vi "Write Controller Object.vi"(6 "Device Information":T1={"System Hardware Reference"=refnum, "Device Information"={"Resource"="", "Vendor Name"="", "Product Name"="", "Product ID"=0, "Serial Number"="", "Device Class"="", "System Start Time"=timestamp(0 s since 1904-01-01), "Current Time"=timestamp(0 s since 1904-01-01), "Time Zone"="", "Firmware Revision"="", "Image Title"="", "Image Version"="", "System Status"="", "Credential type"=enum."None/Unlocked", "User Added"=FALSE}, "Primary Network Adapter"={"IP Address"="", "MAC Address"="", "IP Address Request Mode"=1, "SubnetMask"="", "Gateway"="", "DNS Server"="", "Adapter Mode"=1, "Adapter Type"=1}, "Secondary Network Adapters"=[]} {"Primary Network Adapter"."IP Address Request Mode" items=["Static"=1, "DHCP/Link Local"=2, "Link-Local Only"=4, "DHCP Only"=8]; "Primary Network Adapter"."Adapter Type" items=["Ethernet"=1, "WLAN"=2]; "Primary Network Adapter"."Adapter Mode" items=["Disabled"=1, "TCP/IP Ethernet"=2, "Deterministic"=4, "EtherCAT"=8, "TCP/IP WLAN Connect"=32, "TCP/IP WLAN Create"=64]; "Secondary Network Adapters"."IP Address Request Mode" items=["Static"=1, "DHCP/Link Local"=2, "Link-Local Only"=4, "DHCP Only"=8]; "Secondary Network Adapters"."Adapter Type" items=["Disabled"=1, "TCP/IP Ethernet"=2, "Deterministic"=4, "EtherCAT"=8, "TCP/IP WLAN Connect"=32, "TCP/IP WLAN Create"=64]; "Secondary Network Adapters"."Adapter Mode" items=["Disabled"=1, "TCP/IP Ethernet"=2, "Deterministic"=4, "EtherCAT"=8, "TCP/IP WLAN Connect"=32, "TCP/IP WLAN Create"=64]; "Device Information"."Product ID" format="%.0x"}, 8 "error in":errorcluster, 9 "Remote Chassis":refnum<class "Chassis.lvclass">[](array[class]), 10 "Local Chassis":refnum<class "Chassis.lvclass">, 11 "Controller in":refnum<class "Controller.lvclass">) -> (0 "error out":errorcluster, 3 "Controller out":refnum<class "Controller.lvclass">)   [LabVIEW 2015, in "SMI.lvlib" / "Controller.lvclass"]
uses:
  Controller.lvclass
  Controls/NetworkDevice.ctl
  Controls/DeviceInformation.ctl
  Controls/NetworkAdapterSettings.ctl
  Chassis/Chassis.lvclass
  Controller.lvclass/Controller.ctl
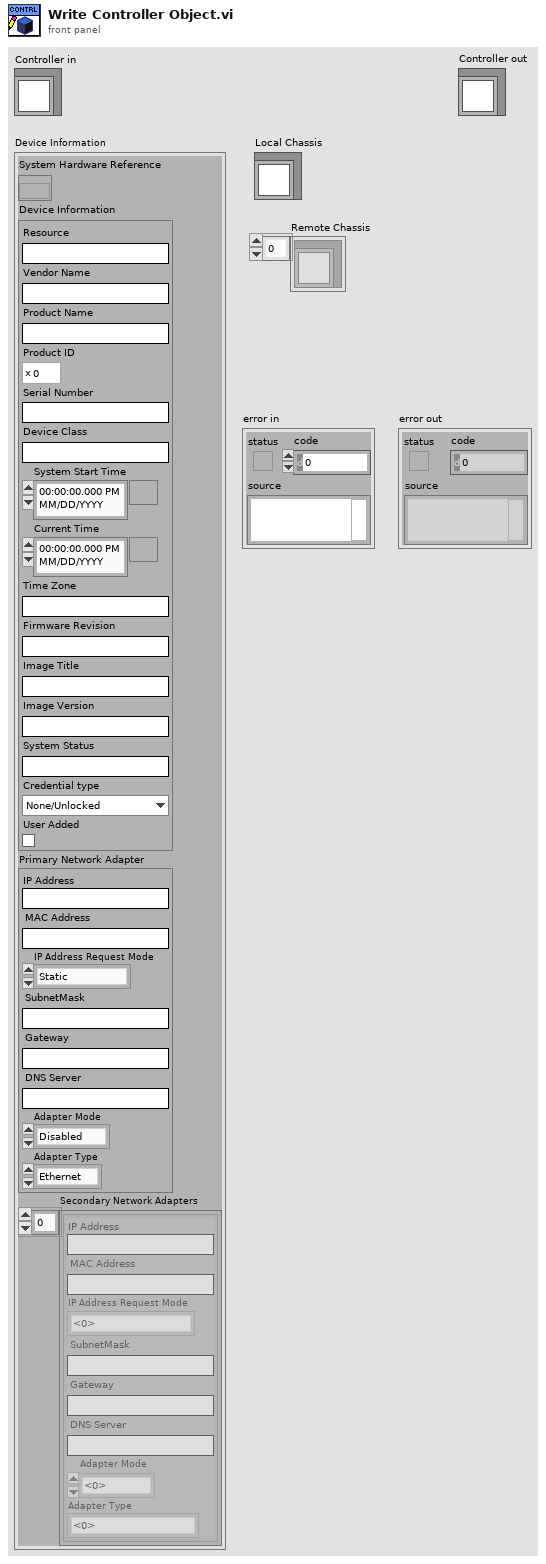
[diagram p1: front panel]
types:
  T1 = typedef "SMI.lvlib/Controller.lvclass/NetworkDevice.ctl" = cluster{"System Hardware Reference":refnum<k20>, "Device Information":T2, "Primary Network Adapter":T3, "Secondary Network Adapters":T3[]}
  T2 = typedef "SMI.lvlib/Controller.lvclass/DeviceInformation.ctl" = cluster{"Resource":string, "Vendor Name":string, "Product Name":string, "Product ID":u32, "Serial Number":string, "Device Class":string, "System Start Time":timestamp, "Current Time":timestamp, "Time Zone":string, "Firmware Revision":string, "Image Title":string, "Image Version":string, "System Status":string, "Credential type":enum16{"None/Unlocked", "FTP Password", "NIAuth Credentials"}, "User Added":bool}
  T3 = typedef "SMI.lvlib/Controller.lvclass/NetworkAdapterSettings.ctl" = cluster{"IP Address":string, "MAC Address":string, "IP Address Request Mode":u32, "SubnetMask":string, "Gateway":string, "DNS Server":string, "Adapter Mode":u32, "Adapter Type":u32}
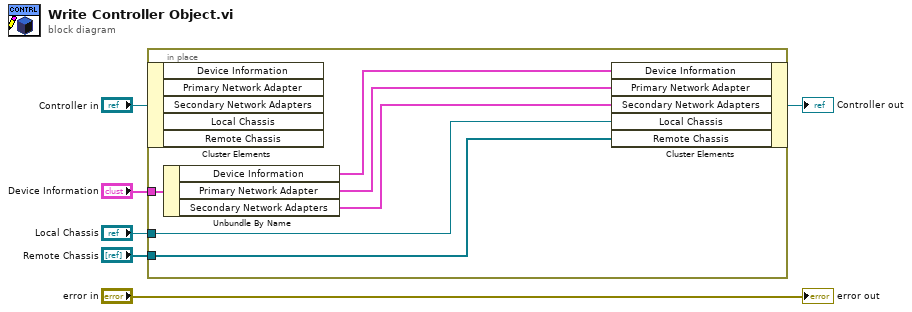
[diagram p0: block diagram]
diagram:
  n1 = in-place {
    in-place-border: "Device Information" -> [w9]
    in-place-border: "Local Chassis" -> [w8]
    in-place-border: "Remote Chassis" -> [w7]
    n2 = in-place-cluster #1("Controller in") -> ()  [unwired: 5 out]
    n3 = Unbundle By Name(w9) -> ("Device Information"=w12:T2, "Primary Network Adapter"=w11:T3, "Secondary Network Adapters"=w10:T3[])
    n4 = in-place-cluster #1("Device Information"=w12, "Primary Network Adapter"=w11, "Secondary Network Adapters"=w10, "Local Chassis"=w8, "Remote Chassis"=w7) -> (→"Controller out":refnum<class "Controller.lvclass">)
  }
  "error out" <- "error in"
